vi "ProjectCode_UsingHardware.vi"() -> ()   [LabVIEW 2023]
uses:
  <vilib>/MakerHub/LINX/Public/Utilities/Open Serial.vi
  <vilib>/MakerHub/LINX/Public/Peripherals/Analog/Analog Read 1 Chan.vi
panel:
  in  "Plant Name":string
  in  "Recipient Email Address:":string
  out "Analog Data":dbl(graph)
  out "Loop Rate (Hz)":u32
  in  "A(n) Channel":u8
  in  "Serial Port":refnum<visa-resource-name>
  out "Time remaining (sec)":i32
  in  "Duration (HOUR[s])":dbl
  out "Time Elapsed (sec)":i32
  in  "Duration (MIN[s])":dbl
  in  "Yes/No":bool
  out "Sensor Output:":dbl
  in  "stop":bool
  out "Plamt Status":T1(ring)
  out "Need to Water?":bool
  # "Email:"
  # "Arduino Parameters:"
  # "<-- Seperate multiple recipients with comma"
  # "Send Additional email reminders?"
  # "How Long to Send Reminder:"
  # "Troubleshooting:"
  # "Reminder Time:"
  # "Sensor Output Graph:"
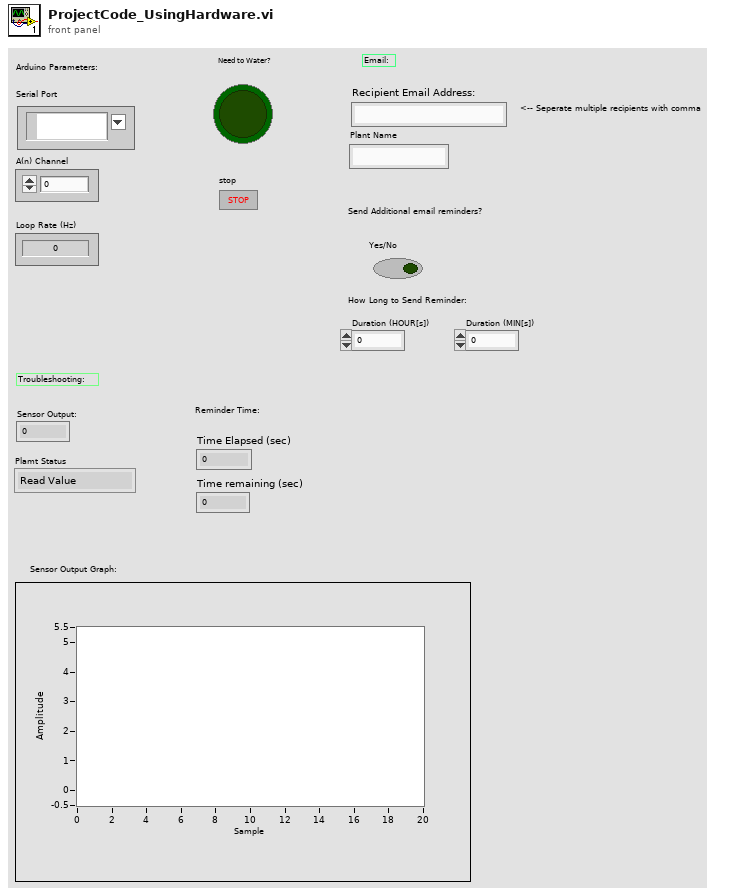
[diagram p1: front panel]
types:
  T1 = enum16{"Read Value", "Send Reminder", "Reminder Timer", "Button Fallbaack"}
  T2 = typedef "LMH-LINX.lvlib/LINX Ref.ctl" = cluster{"IO":T3, "Interface":T4, "LINX Device Config":T5}
  T3 = typedef "LMH-LINX.lvlib/Platform.ctl" = enum16{"Remote", "Local"}
  T4 = typedef "LMH-LINX.lvlib/Interface.ctl" = enum16{"Serial", "TCP"}
  T5 = typedef "LMH-LINX.lvlib/Device.lvlib/LINX Device Config.ctl" = cluster{"Interface":T4, "COM Port":refnum<visa-resource-name>, "TCP Configuration":T6, "Device Family":u8, "Device ID":u8, "Device Name":string, "TCP Ref":refnum<k5>, "Channels":T7}
  T6 = typedef "LMH-LINX.lvlib/Device.lvlib/TCP Config.ctl" = cluster{"IP Address":string, "Port":u16}
  T7 = typedef "LMH-LINX.lvlib/Channels.ctl" = cluster{"DI":u8[], "DO":u8[], "AI":u8[], "AO":u8[], "PWM":u8[], "QE":u8[], "UART":u8[], "I2C 2":u8[], "SPI":u8[], "CAN":u8[], "Servo":u8[], "AI Ref (V)":dbl, "AI Resolution (Bits)":u8, "AO Ref (V)":dbl, "AO Resolution (Bits)":u8}
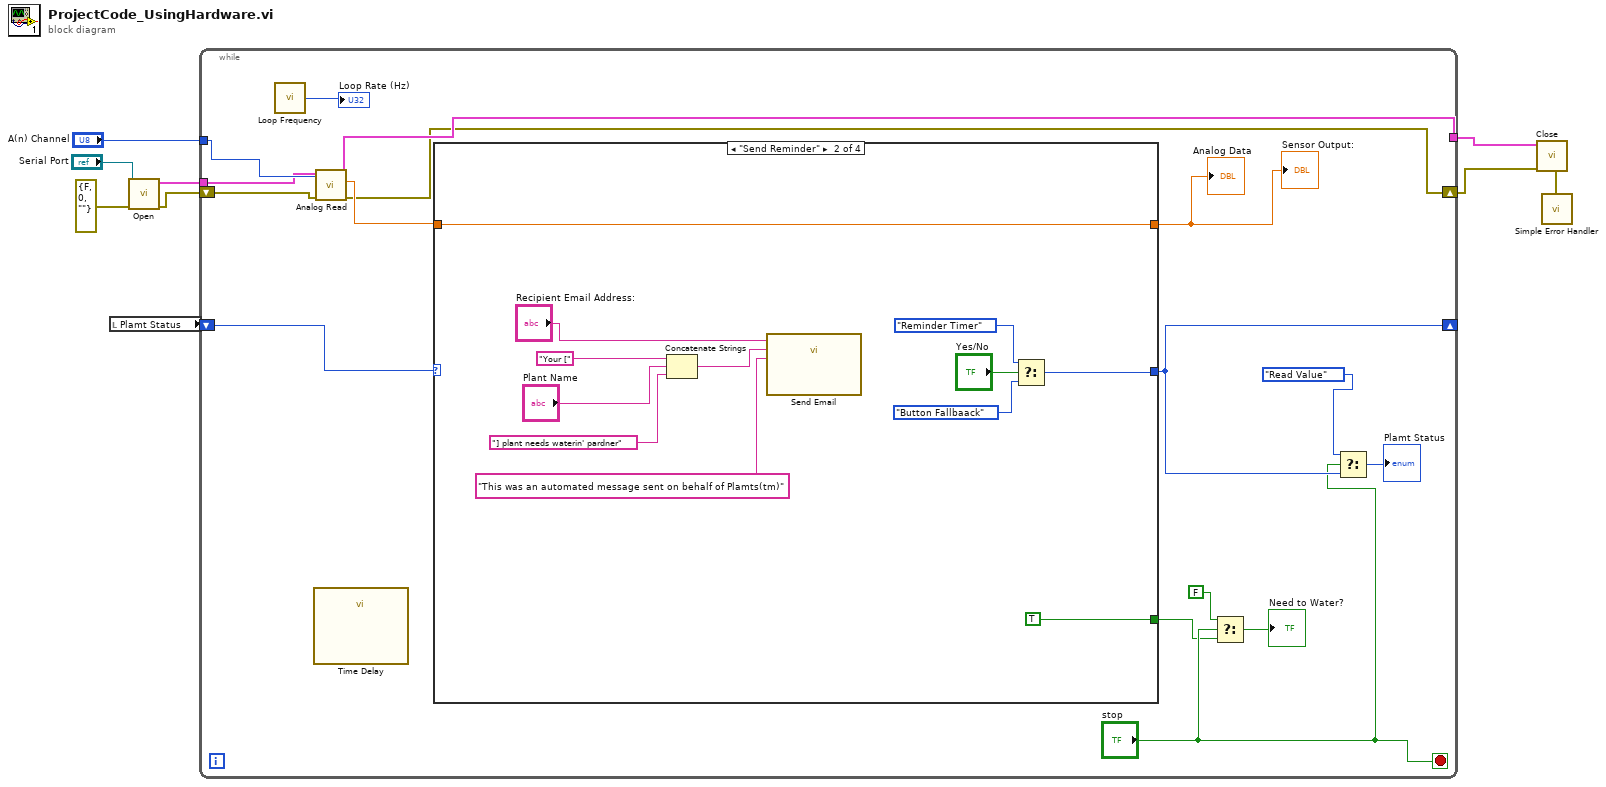
[diagram p0: block diagram]
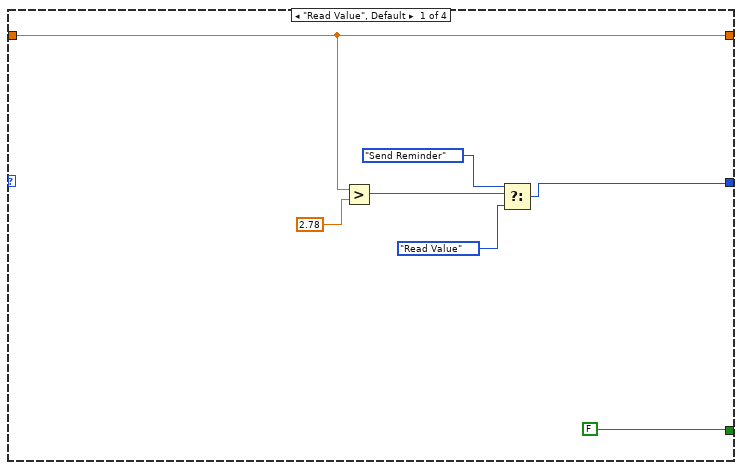
[diagram p2: hidden frame]
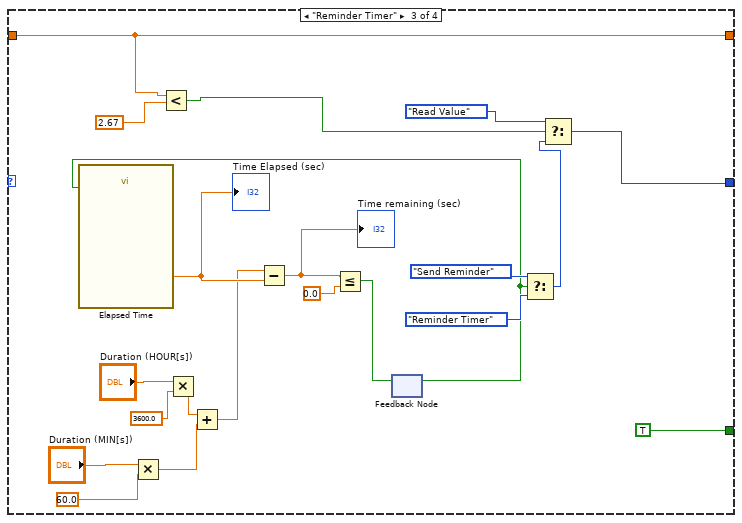
[diagram p3: hidden frame]
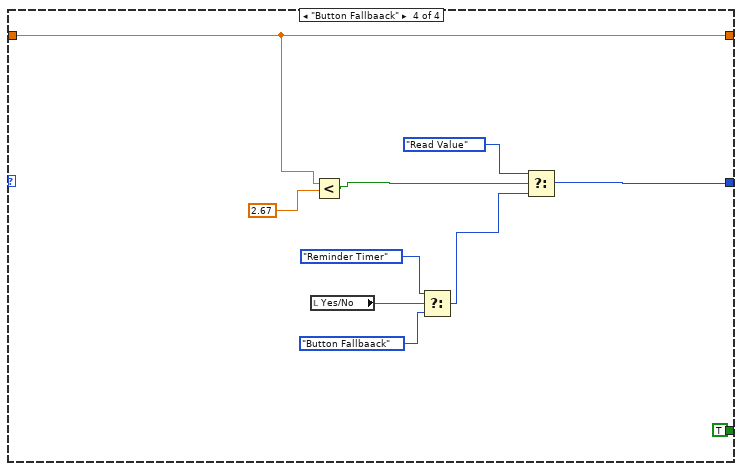
[diagram p4: hidden frame]
diagram:
  n1 = local read "Plamt Status"() -> (w9:T1)
  n2 = call-poly <vilib>:"Open.vi"("Error In"=errorcluster {"status"=FALSE, "code"=0, "source"=""}, "Serial Port"="Serial Port") -> ("Error Out"=w4:errorcluster, "LINX Resource"=w6:T2)  [unwired: 7 in, 1 out]
  n3 = while {
    shift-right: [w24] -> _
    shift-left: w9 -> [w23]
    tunnel: "A(n) Channel" -> [w20]
    tunnel: w6 -> [w19]
    tunnel: [w15] -> w2
    shift-right: [w14] -> w1
    shift-left: w4 -> [w16]
    stop <- "stop" stop-if-true
    n4 = call <vilib>:"Loop Frequency.vi"() -> ("Loop Rate (Hz)"=→"Loop Rate (Hz)":u32)
    n5 = call "Time Delay"() -> ()  [unwired: 11 in, 1 out]
    n6 = call-poly <vilib>:"Analog Read.vi"("Error In"=w16, "Analog Channel"=w20, "LINX Resource"=w19) -> ("Error Out"=w14:errorcluster, "Voltage"=w21:dbl, "LINX Resource"=w15:T2)  [unwired: 5 in, 1 out]
    n7 = case shown="\"Send Reminder\"" w23 {
      tunnel: w21 -> [w28 w43 w47 w67]
      tunnel: [w30 w42 w52 w74] -> w24
      tunnel: [FALSE TRUE TRUE TRUE] -> w11
      tunnel: [w28 w43 w47 w67] -> w17
      frame "Read Value", Default {
        n8 = Greater?(x=w28, y=2.78) -> (0:w31:bool)
        n9 = Select(t=T1."Send Reminder" ("Plamt Status"), s=w31, f=T1."Read Value" ("Plamt Status")) -> (s? t:f=w30:T1)
      }
      frame "Send Reminder" {
        n10 = Concatenate Strings("Your [", "Plant Name", "] plant needs waterin' pardner") -> (w38:string)
        n11 = call "Send Email"("Message"="This was an automated message sent on behalf of Plamts(tm)", "Subject"=w38, "Recipients"="Recipient Email Address:") -> ()  [unwired: 8 in, 1 out]
        n12 = Select(t=T1."Reminder Timer" ("Plamt Status"), s="Yes/No", f=T1."Button Fallbaack" ("Plamt Status")) -> (s? t:f=w42:T1)
      }
      frame "Reminder Timer" {
        n13 = Multiply(x="Duration (MIN[s])", y=60.0) -> (x*y=w58:dbl)
        n14 = Less?(x=w47, y=2.67) -> (x < y?=w45:bool)
        n15 = Multiply(x="Duration (HOUR[s])", y=3600.0) -> (x*y=w63:dbl)
        n16 = Add(x=w63, y=w58) -> (x+y=w64:dbl)
        n17 = feedback #1() -> (w51:bool)  [unwired: 1 in]
        n18 = call "Elapsed Time"("Reset"=w51) -> ("Elapsed Time (s)"=w65:dbl)  [unwired: 11 in, 7 out]
        "Time Elapsed (sec)" <- w65
        n19 = Subtract(x=w64, y=w65) -> (x-y=w49:dbl)
        "Time remaining (sec)" <- w49
        n20 = Less Or Equal?(x=w49, y=0.0) -> (x <= y?=w48:bool)
        n21 = feedback-in #1(w48) -> ()
        n22 = Select(t=T1."Send Reminder" ("Plamt Status"), s=w51, f=T1."Reminder Timer" ("Plamt Status")) -> (s? t:f=w54:T1)
        n23 = Select(t=T1."Read Value" ("Plamt Status"), s=w45, f=w54) -> (s? t:f=w52:T1)
      }
      frame "Button Fallbaack" {
        n24 = local read "Yes/No"() -> (w69:bool)
        n25 = Less?(x=w67, y=2.67) -> (x < y?=w66:bool)
        n26 = Select(t=T1."Reminder Timer" ("Plamt Status"), s=w69, f=T1."Button Fallbaack" ("Plamt Status")) -> (s? t:f=w70:T1)
        n27 = Select(t=T1."Read Value" ("Plamt Status"), s=w66, f=w70) -> (s? t:f=w74:T1)
      }
    }
    "Sensor Output:" <- w17
    "Analog Data" <- w17
    n28 = Select(t=FALSE, s="stop", f=w11) -> (s? t:f=→"Need to Water?":bool)
    n29 = Select(t=T1."Read Value" ("Plamt Status"), s="stop", f=w24) -> (s? t:f=→"Plamt Status":T1)
  }
  n30 = call <vilib>:"Close.vi"("Error In"=w1, "LINX Resource"=w2) -> ("Error Out"=w3:errorcluster)  [unwired: 9 in]
  n31 = call <vilib>:"Simple Error Handler.vi"("error in (no error)"=w3) -> ()  [unwired: 4 in, 5 out]
